vi "New Project.vi"(8 "error in":errorcluster, 11 "Projects":refnum<class "Projects.lvclass">) -> (0 "error out":errorcluster, 3 "Projects out":refnum<class "Projects.lvclass">)   [LabVIEW 2020, in "Main_Process.lvlib"]
doc: "Define a new project and the tasks that should be included with it."
uses:
  Main_Process.lvlib
  Projects/Parent/Projects.lvclass
panel:
  in  "Cancel":bool
  in  "OK":bool
  in  "Tasks":string[](array[string])
  in  "Default Tasks":bool=TRUE
  in  "New Project Name":string
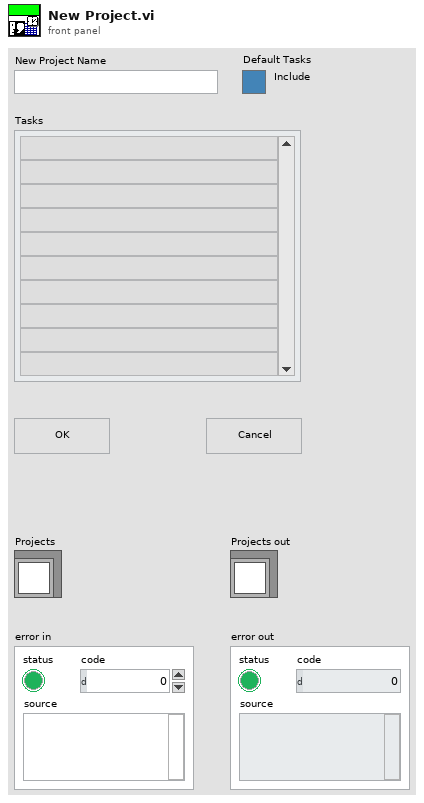
[diagram p1: front panel]
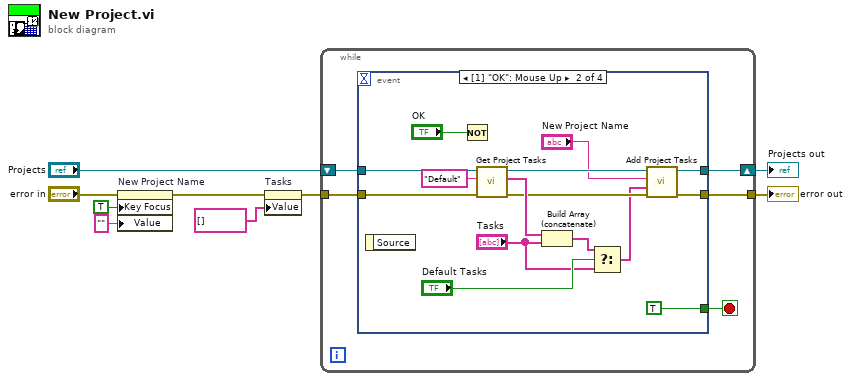
[diagram p0: block diagram]
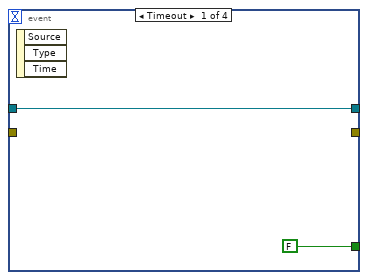
[diagram p2: hidden frame]
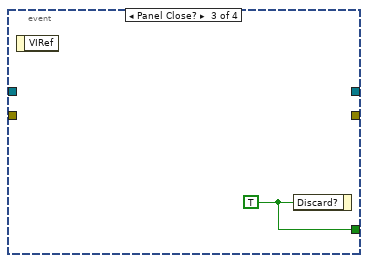
[diagram p3: hidden frame]
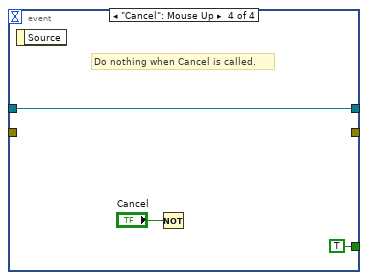
[diagram p4: hidden frame]
diagram:
  n1 = property on="New Project Name" class="Str"(error in="error in", "Key Focus"=TRUE, "Value"="" ("New Project Name")) -> (error out=w3:errorcluster)  [unwired: 1 in, 1 out]
  n2 = property on="Tasks" class="Arr (strict)"(error in=w3, "Value"=string[] [] ("Tasks")) -> (error out=w2:errorcluster)  [unwired: 1 in, 1 out]
  n3 = while {
    shift-right: [w12] -> w8
    shift-left: "Projects" -> [w14]
    tunnel: w2 -> [w11]
    tunnel: [w10] -> w7
    stop <- w13 stop-if-true
    n4 = event shown="[1] \"OK\": Mouse Up" {
      selector: _ -> [_ _ _ _]
      dyn-events: _ -> [_ _ _ _]
      timeout: _ -> [_ _ _ _]
      tunnel: w14 -> [w15 w31 _ w34]
      tunnel: [FALSE TRUE ("Discard?") w32 TRUE ("Discard?")] -> w13
      tunnel: [w15 w20 _ w34] -> w12
      tunnel: w11 -> [_ w29 _ _]
      tunnel: [_ w19 _ _] -> w10
      event Timeout {
        n5 = event-data() -> ()  [unwired: 1 in, 3 out]
      }
      event "OK": Mouse Up {
        n6 = event-data() -> ()  [unwired: 1 in, 1 out]
        n7 = Not(x="OK") -> ()  [unwired: 1 out]
        n8 = call-dynamic "Get Project Tasks.vi"("error in (no error)"=w29, "Project Name"="Default", "Projects in"=w31) -> ("error out"=w23:errorcluster, "Tasks"=w28:string[], "Projects out"=w24:refnum<class "Projects.lvclass">)  [unwired: 6 in]
        n9 = Build Array (concatenate)(w28, "Tasks") -> (w26:string[])
        n10 = Select(t=w26, s="Default Tasks", f="Tasks") -> (s? t:f=w21:string[])
        n11 = call-dynamic "Add Project Tasks.vi"("error in (no error)"=w23, "Tasks"=w21, "Project Name"="New Project Name", "Projects in"=w24) -> ("error out"=w19:errorcluster, "Projects out"=w20:refnum<class "Projects.lvclass">)  [unwired: 5 in, 1 out]
      }
      event Panel Close? {
        w32 = TRUE ("Discard?")
        n12 = event-data() -> ()  [unwired: 1 in, 1 out]
        n13 = event-data("Discard?"=w32) -> ()  [unwired: 1 in, 1 out]
      }
      event "Cancel": Mouse Up {
        # "Do nothing when Cancel is called."
        n14 = event-data() -> ()  [unwired: 1 in, 1 out]
        n15 = Not(x="Cancel") -> ()  [unwired: 1 out]
      }
    }
  }
  "Projects out" <- w8
  "error out" <- w7
